vi "Test Intensity Graph.vi"() -> ()   [LabVIEW 2014]
panel:
  out "min value":dbl
  out "max value":dbl
  out "Intensity Graph":dbl[][](graph)
  out "size(s)":i32
  in  "Custom Marker Colors":u32[](array[colorbox])=[16714752, 16748562, 16773418]
  in  "Array":dbl[][](array[numeric])=[[222.8, 222.8, 222.8, 221.0, 0.0], [220.2, 220.7, 221.6, 222.2, 222.3], [222.4, 222.4, 222.4, 222.5, 0.0], [222.5, 222.5, 222.5, 222.5, 222.5], [0.0, 0.0, 0.0, 0.0, 0.0]]
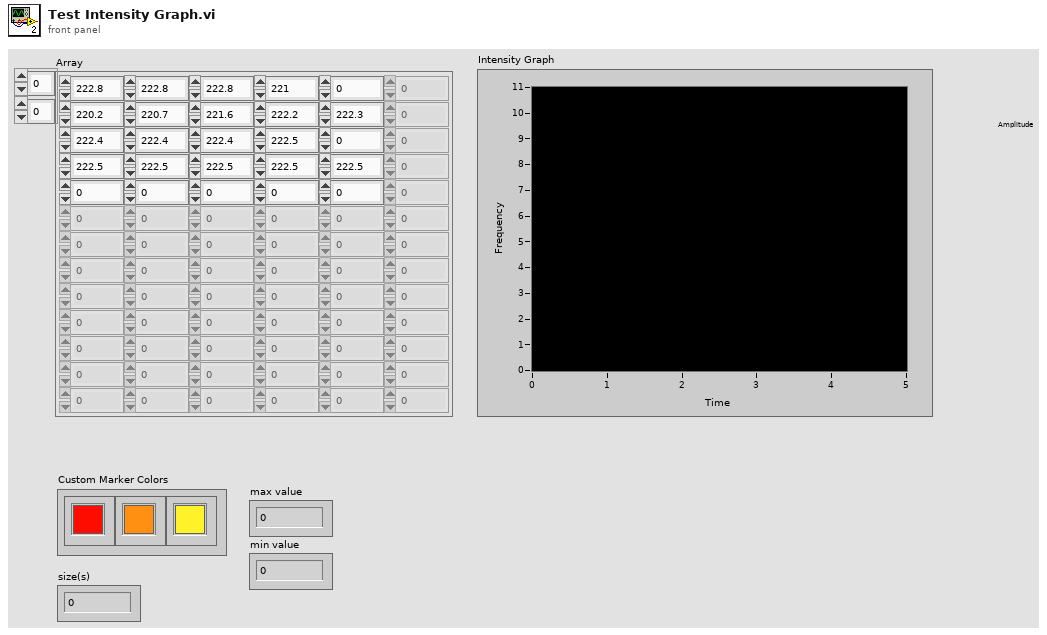
[diagram p1: front panel]
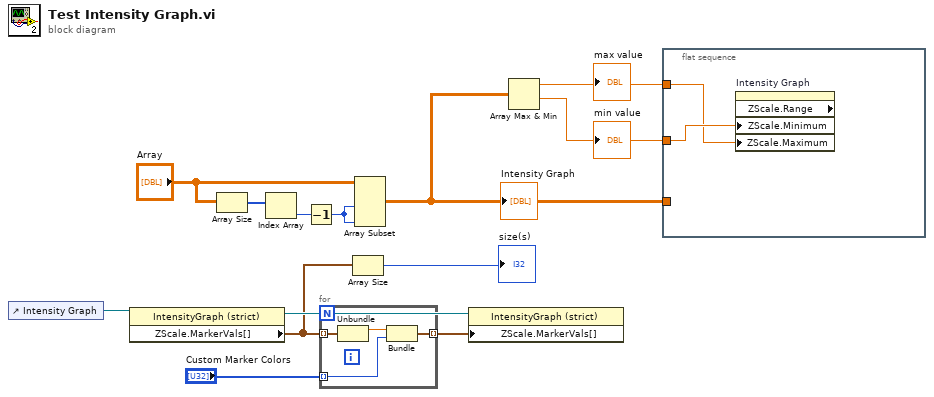
[diagram p0: block diagram]
diagram:
  n1 = control-ref of="Intensity Graph"() -> (w4:refnum<vi>)
  n2 = property on="Property Node" class="IntensityGraph (strict)"(reference=w4) -> (reference out=w7:refnum<vi>, "ZScale.MarkerVals[]"=w6:cluster{dbl, u32}[])  [unwired: 1 in, 1 out]
  n3 = Array Size(array="Array") -> (size(s)=w13:i32[])
  n4 = Index Array(array=w13) -> (element=w12:i32)  [unwired: 1 in]
  n5 = Decrement(x=w12) -> (x-1=w11:i32)
  n6 = for {
    tunnel: w6 -> [w17] mode=indexing
    tunnel: "Custom Marker Colors" -> [w15] mode=indexing
    tunnel: [w14] -> w8 mode=indexing
    n7 = Unbundle(w17) -> (w16:dbl)  [unwired: 1 out]
    n8 = Bundle(w16, "Color Box"=w15) -> (w14:cluster{dbl, "Color Box":u32})  [unwired: 1 in]
  }
  n9 = Array Size(array=w6) -> (size(s)=→"size(s)":i32)
  n10 = Array Subset(array="Array", length (row)=w11, length (col)=w11) -> (w3:dbl[][])  [unwired: 2 in]
  "Intensity Graph" <- w3
  n11 = property on="Property Node" class="IntensityGraph (strict)"(reference=w7, "ZScale.MarkerVals[]"=w8) -> ()  [unwired: 1 in, 2 out]
  n12 = Array Max & Min(array=w3) -> (max value=w1:dbl, min value=w2:dbl)  [unwired: 2 out]
  "max value" <- w1
  "min value" <- w2
  n13 = flat-sequence {
    tunnel: w3 -> [_]
    tunnel: w2 -> [w19]
    tunnel: w1 -> [w18]
    frame #0 {
      n14 = property on="Intensity Graph" class="IntGraph (strict)" props=["ZScale", "Range", "ZScale", "Minimum", "ZScale", "Maximum"]("ZScale.Minimum"=w19, "ZScale.Maximum"=w18) -> ()  [unwired: 2 in, 3 out]
    }
  }
